vi "TestFillState.vi"(8 "Error In":errorcluster, 10 "Module No":i16, 11 "DLL Path":path) -> (0 "Error Out":errorcluster, 2 "Module No":i16, 3 "DLL Path":path)   [LabVIEW 2017]
doc: "This VI is a wrapper for the 'SPC_test_state.vi' checking the flag 'SPC_HFILL_NRDY' in a loop till it becomes inactive or a timeout of 25sec occurs.\nIt is used to wait till the module has finished the filling process initiated by SPC_fill_memory.vi.\n\n<b>Note:</b> This VI is set to execute as preallocated clone to improve performance when run in parallel loops for multi module setups.\n\ninfo@becker-hickl.com"
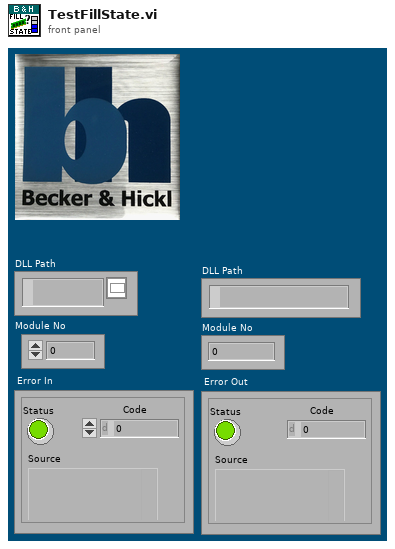
[diagram p1: front panel]
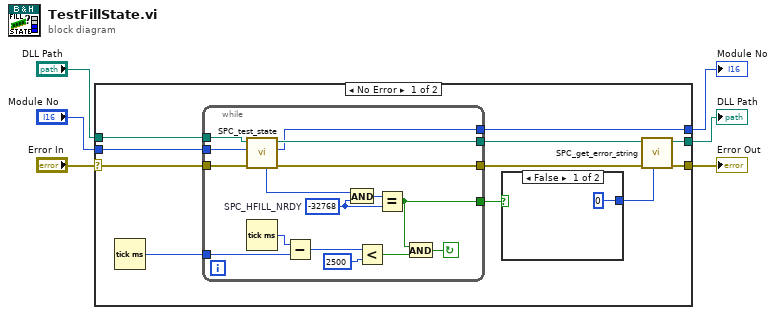
[diagram p0: block diagram]
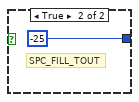
[diagram p2: hidden frame]
diagram:
  n1 = case shown="No Error" "Error In" {
    selector: "Error In" -> [w17 w38]
    tunnel: [w13 w38] -> w6
    tunnel: "DLL Path" -> [w16 w37]
    tunnel: [w12 w37] -> w3
    tunnel: [w8 w36] -> w2
    tunnel: "Module No" -> [w7 w36]
    frame No Error {
      n2 = Tick Count (ms)() -> (millisecond timer value=w10:u32)
      n3 = while {
        tunnel: [w26] -> w9
        tunnel: w10 -> [w31]
        tunnel: w7 -> [w25]
        tunnel: w17 -> [w24]
        tunnel: [w23] -> w14
        tunnel: w16 -> [w22]
        tunnel: [w21] -> w11
        tunnel: [w19] -> w8
        stop <- w33 continue-if-true
        w18 = i16 -32768  # SPC_HFILL_NRDY
        n4 = call "SPC_test_state.vi"("Error In"=w24, "Module No"=w25, "DLL Path"=w22) -> ("Error Out"=w23:errorcluster, "Module No"=w19:i16, "DLL Path"=w21:path, "State Value"=w20:i16)  [unwired: 5 in]
        n5 = Tick Count (ms)() -> (millisecond timer value=w32:u32)
        n6 = Subtract(x=w32, y=w31) -> (x-y=w30:u32)
        n7 = And(x=w20, y=w18) -> (x .and. y?=w27:i16)
        n8 = Less?(x=w30, y=u32 2500) -> (x < y?=w28:bool)
        n9 = Equal?(x=w27, y=w18) -> (x = y?=w26:bool)
        n10 = And(x=w26, y=w28) -> (x .and. y?=w33:bool)
      }
      n11 = case shown="False" w9 {
        tunnel: [i16 0 i16 -25] -> w15
        frame False {
        }
        frame True {
          # "SPC_FILL_TOUT"
        }
      }
      n12 = call "SPC_get_error_string.vi"("ErrorID"=w15, "Error In"=w14, "DLL Path"=w11) -> ("Error Out"=w13:errorcluster, "DLL Path"=w12:path)  [unwired: 6 in, 1 out]
    }
    frame Error {
    }
  }
  "Error Out" <- w6
  "DLL Path" <- w3
  "Module No" <- w2
